vi "ma_sml_Cascaded Decimation Filter (complex input).vi"(1 "reset?":bool, 2 "filter specification":cluster{"h":dbl[], "M":i32, "N":i32}={"h"=[5.017842402298822e-06, -3.6347034460970388e-06, -1.3387466661726196e-05, -7.845024922393745e-07, 2.4426233326325416e-05, 1.069359798524219e-05, -3.953063749330246e-05, -3.449004233474014e-05, 5.166753079423074e-05, 7.580241145008019e-05, -5.202393998060288e-05, -0.00013695088647737978, 2.644152675547298e-05, 0.00021368550203212212, 4.161120271313457e-05, -0.00029287162186333453, -0.00016800576540118464, 0.0003500423446652448, 0.0003622558258869545, -0.0003494082460775069, -0.0006207716924522643, 0.0002469255850065727, 0.0009198920769782536, 2.737152974592998e-06, -0.0012106430242707475, -0.0004354608386366535, 0.0014171861215696209, 0.0010641089924028914, -0.0014408790456388381, -0.0018642019842870067, 0.0011711992096026893, 0.0027616563661223034, -0.0005036324432956759, -0.0036258957001366787, -0.0006367796558850806, 0.00427135221964554, 0.0022690471070142635, -0.00446945340095769, -0.004330934234499924, 0.00397160860790426, 0.006659262862425487, -0.0025415780984074064, -0.008979784594616836, -6.458801396183972e-06, 0.010908888620151816, 0.0037696314078308054, -0.011966313250411517, -0.008724382417252324, 0.01159298865991561, 0.01470707822463853, -0.009159906105557362, -0.021412246936221454, 0.003936970653343424, 0.02841100284536082, 0.005054265927768018, -0.035189042115008715, -0.01953602497219576, 0.0412002318343485, 0.043765506251261, -0.04592888866554608, -0.09358505861942605, 0.048951961493948204, 0.3140370477958766, 0.45000812179125654, 0.3140370477958766, 0.048951961493948204, -0.09358505861942605, -0.04592888866554608, 0.043765506251261, 0.0412002318343485, -0.01953602497219576, -0.035189042115008715, 0.005054265927768018, 0.02841100284536082, 0.003936970653343424, -0.021412246936221454, -0.009159906105557362, 0.01470707822463853, 0.01159298865991561, -0.008724382417252324, -0.011966313250411517, 0.0037696314078308054, 0.010908888620151816, -6.458801396183972e-06, -0.008979784594616836, -0.0025415780984074064, 0.006659262862425487, 0.00397160860790426, -0.004330934234499924, -0.00446945340095769, 0.0022690471070142635, 0.00427135221964554, -0.0006367796558850806, -0.0036258957001366787, -0.0005036324432956759, 0.0027616563661223034, 0.0011711992096026893, -0.0018642019842870067, -0.0014408790456388381, 0.0010641089924028914, 0.0014171861215696209, -0.0004354608386366535, -0.0012106430242707475, 2.737152974592998e-06, 0.0009198920769782536, 0.0002469255850065727, -0.0006207716924522643, -0.0003494082460775069, 0.0003622558258869545, 0.0003500423446652448, -0.00016800576540118464, -0.00029287162186333453, 4.161120271313457e-05, 0.00021368550203212212, 2.644152675547298e-05, -0.00013695088647737978, -5.202393998060288e-05, 7.580241145008019e-05, 5.166753079423074e-05, -3.449004233474014e-05, -3.953063749330246e-05, 1.069359798524219e-05, 2.4426233326325416e-05, -7.845024922393745e-07, -1.3387466661726196e-05, -3.6347034460970388e-06, 5.017842402298822e-06], "M"=2, "N"=0} {"h" format="%.2f"}, 3 "x":cdb[](array[numeric]) format="%.2f") -> (0 "y":cdb[](array[numeric]) format="%.2f")   [LabVIEW 2020, in "NI_MAPro.lvlib"]
doc: "This function filters input signal x and then decimates the output by M^N. It is equal to N stage of decimation by M filter. Each of the decimation by M filter has the same filter coefficients."
uses:
  NI_MAPro.lvlib
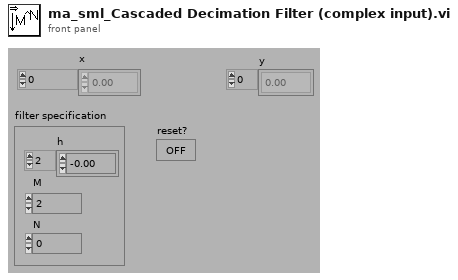
[diagram p1: front panel]
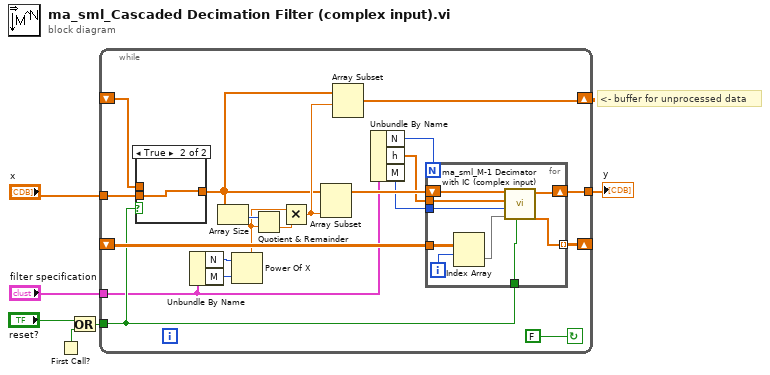
[diagram p0: block diagram]
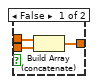
[diagram p2: hidden frame]
diagram:
  # "<- buffer for unprocessed data"
  n1 = First Call?() -> (First Call?: T/F=w2:bool)
  n2 = Or(x="reset?", y=w2) -> (x .or. y?=w3:bool)
  n3 = while {
    tunnel: "filter specification" -> [w7]
    tunnel: w3 -> [w9]
    tunnel: [w11] -> w5
    tunnel: "x" -> [w23]
    shift-left: _ -> [w24]
    shift-right: [w10] -> _
    shift-left: _ -> [w25]
    shift-right: [w26] -> _
    stop <- FALSE continue-if-true
    n4 = case shown="True" w9 {
      tunnel: w24 -> [w29 _]
      tunnel: w23 -> [w28 w30]
      tunnel: [w27 w30] -> w17
      frame False {
        n5 = Build Array (concatenate)(w29, w28) -> (w27:cdb[])
      }
      frame True {
      }
    }
    n6 = Unbundle By Name(w7) -> ("N"=w21:i32, "M"=w20:i32)
    n7 = Array Size(array=w17) -> (size(s)=w22:i32)
    n8 = Power Of X(1:w20, 2:w21) -> (0:w12:dbl)
    n9 = Quotient & Remainder(x=w22, y=w12) -> (floor(x/y)=w13:dbl)  [unwired: 1 out]
    n10 = Multiply(x=w12, y=w13) -> (x*y=w18:dbl)
    n11 = Array Subset(array=w17, length=w18) -> (w19:cdb[])  [unwired: 1 in]
    n12 = Array Subset(array=w17, index=w18) -> (w10:cdb[])  [unwired: 1 in]
    n13 = Unbundle By Name(w7) -> ("N"=w16:i32, "h"=w14:dbl[], "M"=w15:i32)
    n14 = for {
      N: w16 -> [_]
      tunnel: [w39] -> w26 mode=indexing
      tunnel: w25 -> [w33]
      tunnel: w15 -> [w38]
      shift-right: [w36] -> w11
      shift-left: w19 -> [w37]
      tunnel: w14 -> [w32]
      tunnel: w9 -> [w31]
      i -> [w34]
      n15 = Index Array(array=w33, index (row)=w34) -> (element=w35:cdb[])  [unwired: 1 in]
      n16 = call "ma_sml_M-1 Decimator with IC (complex input).vi"("x"=w37, "coefficients"=w32, "M"=w38, "initial conditions"=w35, "reset?"=w31) -> ("y"=w36:cdb[], "final conditions"=w39:cdb[])
    }
  }
  "y" <- w5
